vi "config daq.vi"(0 "task in":refnum<k21>, 1 "Server Method":T2={"scan rate (Hz)"=100.0, "Channel group array"=[], "Number of groups"=1} {"Number of groups" min=1; "Channel group array"."max voltage" format="%.4f"; "scan rate (Hz)" format="%.2f"}) -> (7 "task out":refnum<k21>, 8 "Server Stats":T1={"scan rate"=10.0, "# connections"=0, "channel settings"=[]} {"channel settings"."lower input limits" format="%.4f"; "channel settings"."upper input limits" format="%.4f"; "scan rate" format="%.2f"})   [LabVIEW 2012]
uses:
  Dataserver method.ctl
  Server stats.ctl
  <vilib>/DAQmx/create/channels.llb/DAQmx Create Channel (AI-Voltage-Basic).vi
  <vilib>/DAQmx/configure/timing.llb/DAQmx Timing (Sample Clock).vi
  <resource>/objmgr/daqmx.rc
panel:
  out "channels per group":u32[](array[numeric])
  out "Channels":refnum<k21>[](array[refnum])
  out "NumChans":u32
  out "error out":errorcluster
  # "Hz"
  # "Hz"
  # "channel identifiers"
  # "max voltage"
  # "port locations"
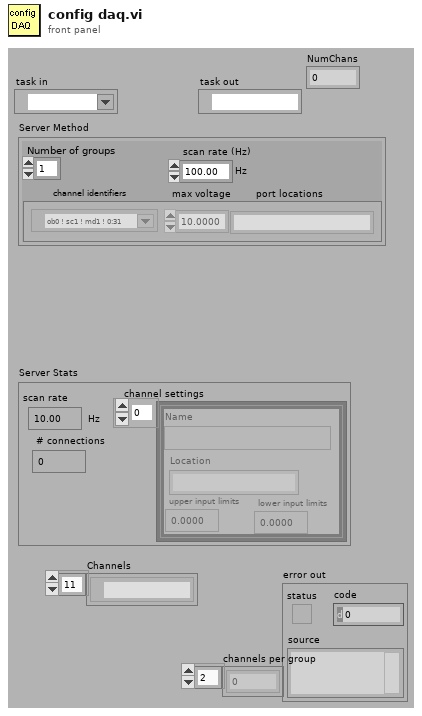
[diagram p1: front panel]
types:
  T1 = typedef "Server stats.ctl" = cluster{"scan rate":dbl, "# connections":i32, "channel settings":cluster{"Name":string, "upper input limits":sgl, "lower input limits":sgl, "Location":string}[]}
  T2 = typedef "Dataserver method.ctl" = cluster{"scan rate (Hz)":dbl, "Channel group array":cluster{"channels":tag, "max voltage":sgl, "Port locations":string}[], "Number of groups":u8}
  T3 = cluster{"channels":tag, "max voltage":sgl, "Port locations":string}[]
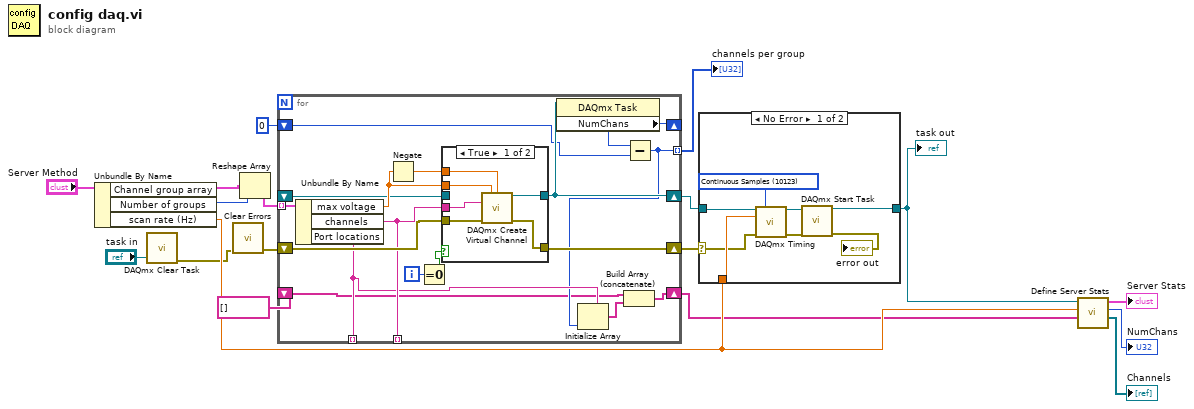
[diagram p0: block diagram]
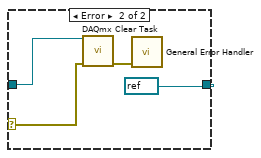
[diagram p2: hidden frame]
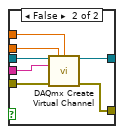
[diagram p3: hidden frame]
diagram:
  n1 = Unbundle By Name("Server Method") -> ("Channel group array"=w14:T3, "Number of groups"=w13:u8, "scan rate (Hz)"=w16:dbl)
  n2 = call <vilib>:"DAQmx Clear Task.vi"("task in"="task in") -> ("error out"=w10:errorcluster)  [unwired: 14 in]
  n3 = call <vilib>:"Clear Errors.vi"("error in (no error)"=w10) -> ("error out"=w15:errorcluster)  [unwired: 6 in]
  n4 = Reshape Array(w14, w13) -> (w18:T3)
  n5 = for {
    tunnel: w18 -> [w27] mode=indexing
    tunnel: [w23] -> _ mode=indexing
    shift-right: [w26] -> w9
    shift-left: _ -> [w29]
    shift-right: [w33] -> w17
    shift-left: w15 -> [w32]
    tunnel: [w31] -> _ mode=indexing
    tunnel: [w22] -> w7 mode=indexing
    shift-right: [w25] -> _
    shift-left: u32 0 ("NumChans") -> [w24]
    shift-right: [w21] -> w5
    shift-left: string[] [] -> [w19]
    i -> [w30]
    n6 = Unbundle By Name(w27) -> ("max voltage"=w34:sgl, "channels"=w31:tag, "Port locations"=w23:string)
    n7 = Negate(x=w34) -> (-x=w35:sgl)
    n8 = Equal To 0?(x=w30) -> (x = 0?=w28:bool)
    n9 = case shown="True" w28 {
      tunnel: w35 -> [w41 w48]
      tunnel: w34 -> [w40 w47]
      tunnel: [w39 w46] -> w26
      tunnel: [w38 w45] -> w33
      tunnel: w32 -> [w37 w44]
      tunnel: w31 -> [w36 w43]
      tunnel: w29 -> [_ w42]
      frame True {
        n10 = call-poly <vilib>:"DAQmx Create Virtual Channel.vi"("maximum value"=w40, "minimum value"=w41, "physical channels"=w36, "error in"=w37) -> ("task out"=w39:refnum<k21>, "error out"=w38:errorcluster)  [unwired: 10 in]
      }
      frame False {
        n11 = call-poly <vilib>:"DAQmx Create Virtual Channel.vi"("task in"=w42, "maximum value"=w47, "minimum value"=w48, "physical channels"=w43, "error in"=w44) -> ("task out"=w46:refnum<k21>, "error out"=w45:errorcluster)  [unwired: 9 in]
      }
    }
    n12 = property class="DAQmx Task"(reference=w26) -> ("NumChans"=w25:u32)  [unwired: 1 in, 2 out]
    n13 = Subtract(x=w25, y=w24) -> (x-y=w22:u32)
    n14 = Initialize Array(w23, w22) -> (w20:string[])
    n15 = Build Array (concatenate)(w19, w20) -> (w21:string[])
  }
  "channels per group" <- w7
  n16 = case shown="No Error" w17 {
    selector: w17 -> [w50 w58]
    tunnel: w9 -> [w55 w60]
    tunnel: [w56 refnum<k21> refnum ("task out")] -> w4
    tunnel: w16 -> [w52 _]
    frame No Error {
      w53 = 10123 items=["Finite Samples"=10178, "Continuous Samples"=10123, "Hardware Timed Single Point"=12522] ("sample mode")
      n17 = call-poly <vilib>:"DAQmx Timing.vi"("task/channels in"=w55, "sample mode"=w53, "rate"=w52, "error in"=w50) -> ("task out"=w54:refnum<k21>, "error out"=w51:errorcluster)  [unwired: 10 in]
      n18 = call <vilib>:"DAQmx Start Task.vi"("task/channels in"=w54, "error in"=w51) -> ("task out"=w56:refnum<k21>, "error out"=→"error out":errorcluster)  [unwired: 12 in]
    }
    frame Error {
      n19 = call <vilib>:"DAQmx Clear Task.vi"("task in"=w60, "error in"=w58) -> ("error out"=w57:errorcluster)  [unwired: 13 in]
      n20 = call <vilib>:"General Error Handler.vi"("error in (no error)"=w57) -> ()  [unwired: 10 in, 5 out]
    }
  }
  "task out" <- w4
  n21 = call "Define Server Stats.vi"("Port locations"=w5, "scan rate (Hz)"=w16, "Refnum in"=w4) -> ("Channels"=→"Channels":refnum<k21>[], "NumChans"=→"NumChans":u32, "Server Stats"=→"Server Stats":T1)  [unwired: 6 in]
